vi "PID Advanced (DBL).vi"(0 "setpoint":dbl format="%.2f", 1 "output range":cluster{"output high":dbl, "output low":dbl}={"output high"=100.0, "output low"=-100.0} {"output low" format="%.2f"; "output high" format="%.2f"}, 2 "auto? (T)":bool=TRUE, 3 "manual control":dbl format="%.2f", 5 "process variable":dbl format="%.2f", 6 "gamma":dbl format="%.2f", 7 "setpoint range":cluster{"setpoint high":dbl, "setpoint low":dbl}={"setpoint high"=100.0, "setpoint low"=0.0} {"setpoint high" format="%.2f"; "setpoint low" format="%.2f"}, 8 "alpha":dbl=nan format="%.2f", 9 "PID gains":T1={"proportional gain (Kc)"=1.0, "integral time (Ti, min)"=0.01, "derivative time (Td, min)"=0.0} {"derivative time (Td, min)" format="%.3f"; "integral time (Ti, min)" format="%.3f"; "proportional gain (Kc)" format="%.3f"}, 11 "dt (s)":dbl=-1.0 format="%.3f", 12 "reinitialize? (F)":bool, 13 "beta":dbl=1.0 format="%.2f", 14 "linearity":dbl=1.0 format="%.2f") -> (4 "output":dbl format="%.2f", 15 "dt out (s)":dbl format="%.3f")   [LabVIEW 2020, in "NI_PID_pid.lvlib"]
doc: "Implements a PID controller using a PID algorithm with advanced optional features. The advanced PID algorithm includes the features of the algorithm the PID VI uses, as well as manual mode control with bumpless manual-to-automatic transitions, nonlinear integral action, two degree-of-freedom control, and error-squared control. Use the DBL instance of this VI to implement a single control loop. Use the DBL Array instance to implement parallel multi-loop control."
uses:
  NI_PID_pid.lvlib
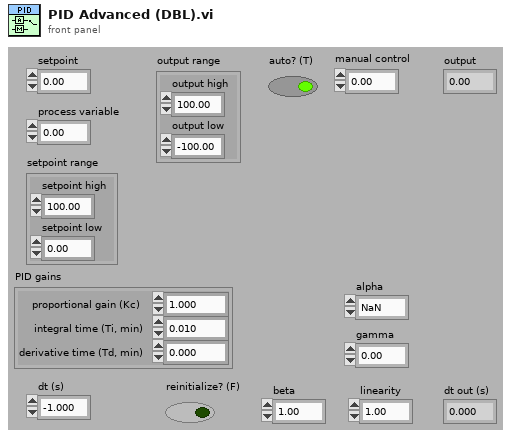
[diagram p1: front panel]
types:
  T1 = cluster{"proportional gain (Kc)":dbl, "integral time (Ti, min)":dbl, "derivative time (Td, min)":dbl}
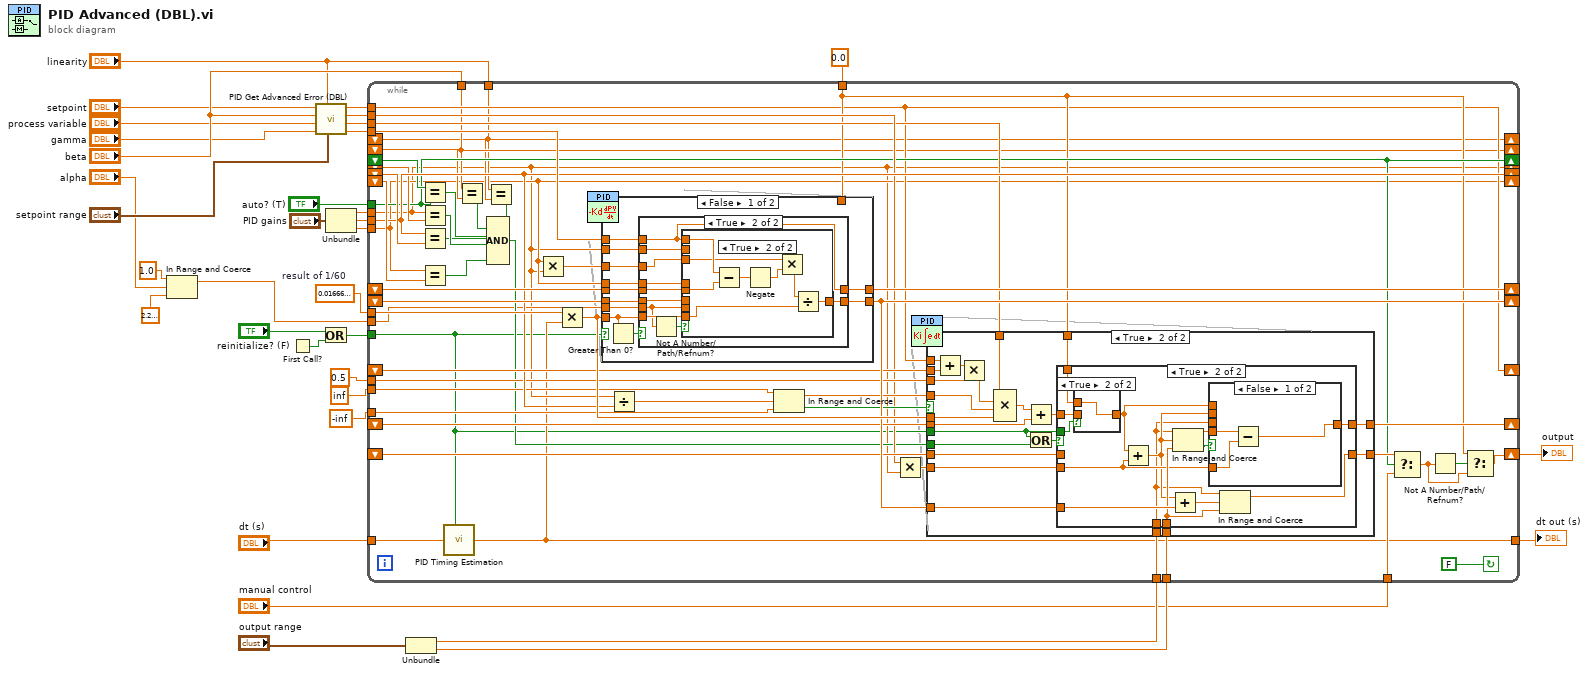
[diagram p0: block diagram]
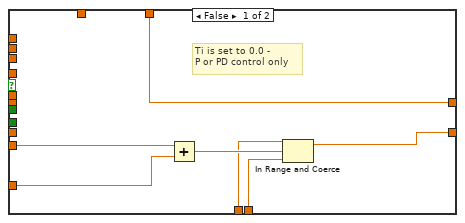
[diagram p2: hidden frame]
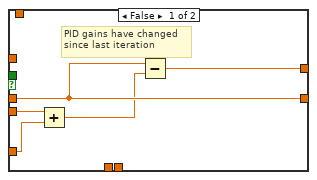
[diagram p3: hidden frame]
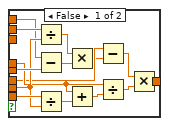
[diagram p7: hidden frame]
diagram:
  w19 = 0.016666666666666666  # result of 1/60
  n1 = In Range and Coerce(upper limit=1.0 ("lower limit"), x="alpha", lower limit=2.220446049250313e-16) -> (coerced(x)=w3:dbl)  [unwired: 1 out]
  n2 = First Call?() -> (First Call?: T/F=w33:bool)
  n3 = call "PID Get Advanced Error (DBL).vi"("setpoint range"="setpoint range", "linearity"="linearity", "Gamma"="gamma", "process variable"="process variable", "beta"="beta", "setpoint"="setpoint") -> ("error with gamma"=w6:dbl, "non-linear integral action"=w13:dbl, "error with beta"=w12:dbl, "error"=w11:dbl)  [unwired: 2 out]
  n4 = Or(x="reinitialize? (F)", y=w33) -> (x .or. y?=w23:bool)
  n5 = Unbundle("PID gains") -> ("proportional gain (Kc)"=w31:dbl, "integral time (Ti, min)"=w30:dbl, "derivative time (Td, min)"=w29:dbl)
  n6 = Unbundle("output range") -> ("output high"=w26:dbl, "output low"=w25:dbl)
  n7 = while {
    tunnel: w23 -> [w35]
    shift-right: [w38] -> _
    shift-left: _ -> [w64]
    shift-right: [w65] -> _
    shift-left: _ -> [w86]
    shift-right: [w39] -> _
    shift-left: _ -> [w87]
    tunnel: w31 -> [w38]
    tunnel: w30 -> [w65]
    tunnel: w29 -> [w39]
    tunnel: "dt (s)" -> [w37]
    tunnel: w26 -> [w82]
    tunnel: w25 -> [w81]
    tunnel: w6 -> [w80]
    shift-right: [w79] -> _
    shift-left: _ -> [w78]
    shift-right: [w77] -> _
    shift-left: _ -> [w70]
    shift-right: [w49] -> w14
    shift-left: _ -> [w76]
    shift-right: [w47] -> _
    shift-left: _ -> [w75]
    shift-right: [w74] -> _
    shift-left: _ -> [w73]
    tunnel: w19 -> [w67]
    tunnel: 0.5 ("y") -> [w63]
    tunnel: inf ("upper limit") -> [w61]
    tunnel: -inf ("lower limit") -> [w62]
    tunnel: w12 -> [w59]
    tunnel: 0.0 ("initial condition") -> [w48]
    tunnel: w13 -> [w58]
    shift-right: [w51] -> _
    shift-left: _ -> [w57]
    tunnel: "auto? (T)" -> [w51]
    tunnel: [w36] -> w16
    tunnel: "manual control" -> [w50]
    tunnel: w11 -> [w47]
    shift-right: [w46] -> _
    shift-left: _ -> [w45]
    tunnel: "beta" -> [w46]
    shift-right: [w43] -> _
    shift-left: _ -> [w41]
    tunnel: "linearity" -> [w43]
    tunnel: w3 -> [w40]
    stop <- FALSE continue-if-true
    n8 = Equal?(x=w57, y=w51) -> (x = y?=w55:bool)
    n9 = Equal?(x=w38, y=w64) -> (x = y?=w84:bool)
    n10 = Equal?(x=w65, y=w86) -> (x = y?=w83:bool)
    n11 = Equal?(x=w39, y=w87) -> (x = y?=w85:bool)
    n12 = call "PID Timing Estimation.vi"("Initialize?"=w35, "dt (s) in"=w37) -> ("dt (s) out"=w36:dbl)  [unwired: 7 in]
    n13 = Equal?(x=w46, y=w45) -> (x = y?=w44:bool)
    n14 = Equal?(x=w43, y=w41) -> (x = y?=w42:bool)
    n15 = Compound Arithmetic op=AND(w42, w44, w55, w84, w83, w85) -> (w56:bool)
    n16 = Multiply(x=w39, y=w38) -> (x*y=w69:dbl)
    n17 = Multiply(x=w67, y=w36) -> (x*y=w88:dbl)
    n18 = case shown="False" w35 {
      tunnel: w78 -> [w153 _]
      tunnel: w69 -> [w150 _]
      tunnel: w80 -> [w152 w190]
      tunnel: [w149 w190] -> w79
      tunnel: [w151 w189] -> w77
      tunnel: w70 -> [w147 _]
      tunnel: w88 -> [w146 _]
      tunnel: w48 -> [_ w189]
      tunnel: w40 -> [w145 _]
      tunnel: w39 -> [w144 _]
      tunnel: w38 -> [w143 _]
      frame False {
        n19 = Greater Than 0?(x=w146) -> (x > 0?=w148:bool)
        n20 = case shown="True" w148 {
          tunnel: w153 -> [w155 w165]
          tunnel: w146 -> [_ w159]
          tunnel: w152 -> [_ w160]
          tunnel: [w154 w164] -> w151
          tunnel: w150 -> [_ w157]
          tunnel: [w155 w160] -> w149
          tunnel: w147 -> [w154 w161]
          tunnel: w145 -> [_ w156]
          tunnel: w144 -> [_ w163]
          tunnel: w143 -> [_ w162]
          frame False {
            # "dt = 0 min"
          }
          frame True {
            n21 = Not A Number/Path/Refnum?(number/path/refnum=w156) -> (NaN/Path/Refnum?=w158:bool)
            n22 = case shown="True" w158 {
              tunnel: w165 -> [w180 w184]
              tunnel: [w179 w185] -> w164
              tunnel: w159 -> [w178 w181]
              tunnel: w156 -> [w177 _]
              tunnel: w163 -> [w176 _]
              tunnel: w162 -> [w175 _]
              tunnel: w161 -> [w174 _]
              tunnel: w160 -> [w166 w183]
              tunnel: w157 -> [_ w182]
              frame False {
                n23 = Divide(x=w175, y=w177) -> (x/y=w171:dbl)
                n24 = Subtract(x=w166, y=w180) -> (x-y=w168:dbl)
                n25 = Divide(x=w178, y=w177) -> (x/y=w173:dbl)
                n26 = Multiply(x=w171, y=w168) -> (x*y=w169:dbl)
                n27 = Add(x=w176, y=w173) -> (x+y=w172:dbl)
                n28 = Subtract(x=w174, y=w169) -> (x-y=w170:dbl)
                n29 = Divide(x=w176, y=w172) -> (x/y=w167:dbl)
                n30 = Multiply(x=w170, y=w167) -> (x*y=w179:dbl)
              }
              frame True {
                n31 = Subtract(x=w183, y=w184) -> (x-y=w188:dbl)
                n32 = Negate(x=w188) -> (-x=w187:dbl)
                n33 = Multiply(x=w182, y=w187) -> (x*y=w186:dbl)
                n34 = Divide(x=w186, y=w181) -> (x/y=w185:dbl)
              }
            }
          }
        }
      }
      frame True {
      }
    }
    n35 = Divide(x=w38, y=w65) -> (x/y=w68:dbl)
    n36 = In Range and Coerce(upper limit=w61, x=w68, lower limit=w62) -> (coerced(x)=w72:dbl, In Range?=w71:bool)
    n37 = Multiply(x=w59, y=w38) -> (x*y=w66:dbl)
    n38 = case shown="True" w71 {
      tunnel: w47 -> [_ w116]
      tunnel: w75 -> [_ w117]
      tunnel: w73 -> [_ w112]
      tunnel: [w89 w107] -> w74
      tunnel: w72 -> [_ w105]
      tunnel: w66 -> [w94 w110]
      tunnel: [w95 w106] -> w52
      tunnel: w76 -> [_ w108]
      tunnel: w77 -> [w93 w104]
      tunnel: w35 -> [_ w103]
      tunnel: w56 -> [_ w102]
      tunnel: w88 -> [_ w101]
      tunnel: w82 -> [w91 w99]
      tunnel: w81 -> [w90 w100]
      tunnel: w63 -> [_ w98]
      tunnel: w48 -> [w89 w97]
      tunnel: w58 -> [_ w96]
      frame False {
        # "Ti is set to 0.0 -\nP or PD control only"
        n39 = Add(x=w94, y=w93) -> (x+y=w92:dbl)
        n40 = In Range and Coerce(upper limit=w91, x=w92, lower limit=w90) -> (coerced(x)=w95:dbl)  [unwired: 1 out]
      }
      frame True {
        n41 = Add(x=w116, y=w117) -> (x+y=w115:dbl)
        n42 = Multiply(x=w115, y=w98) -> (x*y=w114:dbl)
        n43 = Compound Arithmetic op=MULTIPLY(w96, w114, w105, w101) -> (w113:dbl)
        n44 = Add(x=w113, y=w112) -> (x+y=w111:dbl)
        n45 = Or(x=w103, y=w102) -> (x .or. y?=w109:bool)
        n46 = case shown="True" w109 {
          tunnel: w111 -> [_ w130]
          tunnel: w110 -> [w120 w126]
          tunnel: w108 -> [w122 _]
          tunnel: w103 -> [_ w132]
          tunnel: [w121 w128] -> w107
          tunnel: [w122 w135] -> w106
          tunnel: w104 -> [w119 w134]
          tunnel: w100 -> [_ w133]
          tunnel: w99 -> [_ w124]
          tunnel: w97 -> [_ w131]
          frame False {
            # "PID gains have changed\nsince last iteration"
            n47 = Add(x=w120, y=w119) -> (x+y=w118:dbl)
            n48 = Subtract(x=w122, y=w118) -> (x-y=w121:dbl)
          }
          frame True {
            n49 = case shown="True" w132 {
              tunnel: w131 -> [_ w142]
              tunnel: [w141 w142] -> w129
              tunnel: w130 -> [w141 _]
              frame False {
              }
              frame True {
              }
            }
            n50 = Add(x=w129, y=w126) -> (x+y=w125:dbl)
            n51 = Add(x=w125, y=w134) -> (x+y=w136:dbl)
            n52 = In Range and Coerce(upper limit=w124, x=w125, lower limit=w133) -> (coerced(x)=w123:dbl, In Range?=w127:bool)
            n53 = case shown="False" w127 {
              tunnel: w129 -> [_ w140]
              tunnel: [w137 w140] -> w128
              tunnel: w123 -> [w139 _]
              tunnel: w126 -> [w138 _]
              tunnel: w124 -> [_ _]
              tunnel: w125 -> [_ _]
              frame False {
                n54 = Subtract(x=w139, y=w138) -> (x-y=w137:dbl)
              }
              frame True {
              }
            }
            n55 = In Range and Coerce(upper limit=w124, x=w136, lower limit=w133) -> (coerced(x)=w135:dbl)  [unwired: 1 out]
          }
        }
      }
    }
    n56 = Select(t=w52, s=w51, f=w50) -> (s? t:f=w54:dbl)
    n57 = Not A Number/Path/Refnum?(number/path/refnum=w54) -> (NaN/Path/Refnum?=w53:bool)
    n58 = Select(t=w48, s=w53, f=w54) -> (s? t:f=w49:dbl)
  }
  "dt out (s)" <- w16
  "output" <- w14
